vi "Semaphore Lock.vi"(11 "name":string) -> (3 "semaphore":refnum<queue>)   [LabVIEW 2017, in "CSM Shared.lvlib"]
uses:
  CSM Shared.lvlib
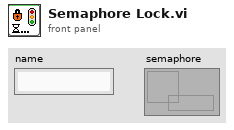
[diagram p1: front panel]
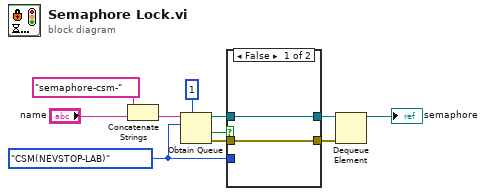
[diagram p0: block diagram]
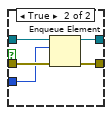
[diagram p2: hidden frame]
diagram:
  w4 = enum16{"CSM(NEVSTOP-LAB)"}."CSM(NEVSTOP-LAB)"
  n1 = Concatenate Strings("semaphore-csm-" ("string"), "name") -> (w2:string)
  n2 = Obtain Queue(max queue size (-1, unlimited)=1, name (unnamed)=w2, element data type=w4) -> (queue out=w8:refnum<queue>, created new?=w6:bool, error out=w9:errorcluster)  [unwired: 2 in]
  n3 = case shown="False" w6 {
    tunnel: [w13 w17] -> w7
    tunnel: w8 -> [w13 w18]
    tunnel: w9 -> [w12 w16]
    tunnel: [w12 w15] -> w10
    tunnel: w4 -> [_ w14]
    frame False {
    }
    frame True {
      n4 = Enqueue Element(queue=w18, element=w14, error in (no error)=w16) -> (queue out=w17:refnum<queue>, error out=w15:errorcluster)  [unwired: 1 in, 1 out]
    }
  }
  n5 = Dequeue Element(queue=w7, error in (no error)=w10) -> (queue out=→"semaphore":refnum<queue>)  [unwired: 1 in, 3 out]
